vi "HeaderAction.vi"(0 "EG_G5210 en entrée":refnum<class "EGG5210.lvclass"> caption="DNL_LabVIEW Object in", 11 "error in (no error)":errorcluster caption="entrée d'erreur (pas d'erreur)") -> (4 "EG_G5210 en sortie":refnum<class "EGG5210.lvclass"> caption="DNL_LabVIEW Object out", 6 "DataNames":string[](array[string]), 8 "Instr Name":string, 10 "HeaderString":string, 14 "DisplayNames":string[](array[string]), 15 "error out":errorcluster caption="sortie d'erreur")   [LabVIEW 2012, in "EGG5210.lvclass"]
uses:
  EGG5210.lvclass
  EGG5210.lvclass/EGG5210.ctl
  <userlib>/EG_G 5210 LIA/ReadFunctions.ctl
  <userlib>/EG_G 5210 LIA/TrigMode.ctl
  BaseDevice/BaseDevice.lvclass
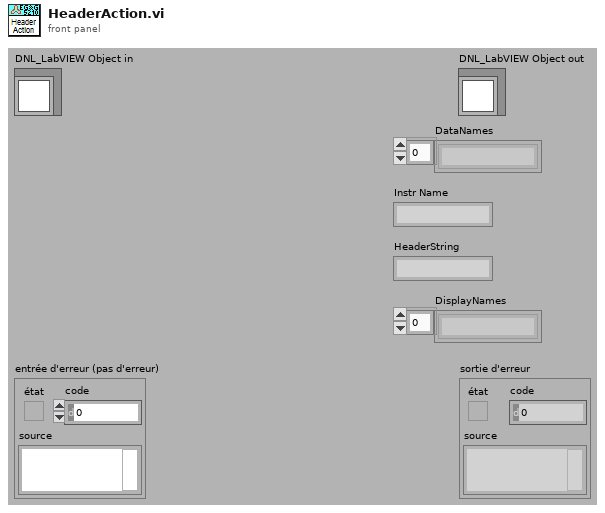
[diagram p1: front panel]
types:
  T1 = typedef "ReadFunctions.ctl" = enum16{"Sensitivity", "Vernier Mode", "Main Filter", "Filter Mode", "Line Filter", "Ref Source", "Ref Mode", "Ref Phase", "Ref Frequency", "Output Filter", "Time Constant", "Dyn Reserve", "X Offset", "Y Offset", "Expand Mode", "Int Oscillator", "Oscillator Freq", "All params", "Overload Byte", "Trigger Mode", "Error"}
  T2 = typedef "EGG5210.lvclass/EGG5210_Func.ctl" = enum16{"Read X & Y (V)", "Read Mag & Phase (V,°)", "Read X, Y, Mag & Phase (V,V,V,°)", "Read ADC Ch1 (V)", "Read ADC Ch2 (V)", "Oscillator Ctrl (Hz, mV rms)", "PL Excimer Settings (Na)"}
  T3 = typedef "TrigMode.ctl" = u16
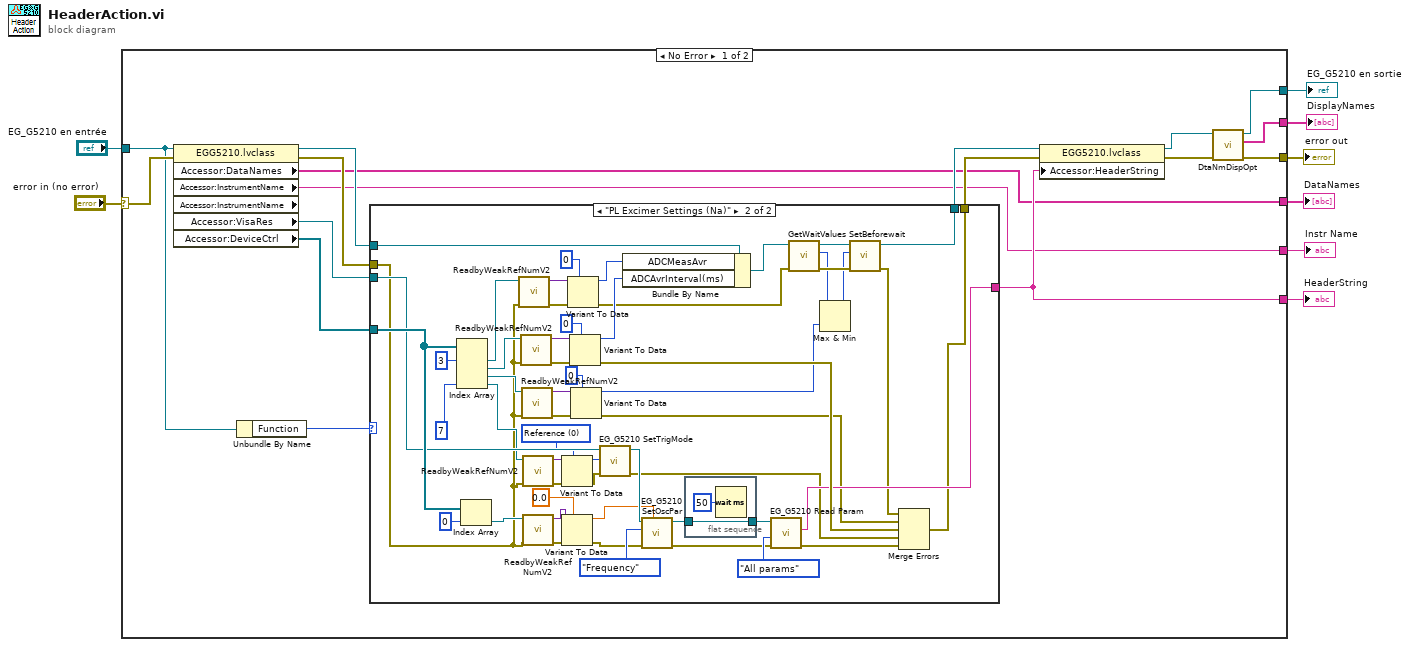
[diagram p0: block diagram]
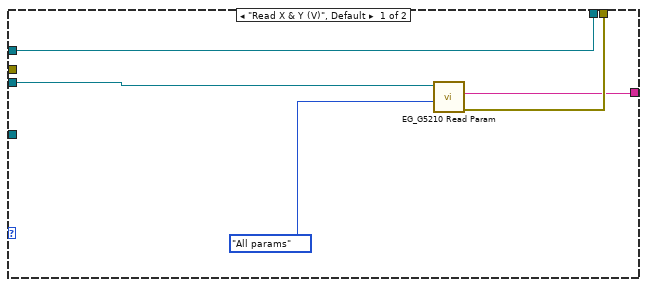
[diagram p2: hidden frame]
diagram:
  n1 = case shown="No Error" "error in (no error)" {
    selector: "error in (no error)" -> [w25 w87]
    tunnel: "EG_G5210 en entrée" -> [w22 w88]
    tunnel: [w10 w88] -> w6
    tunnel: [w15 _] -> w5
    tunnel: [w24 _] -> w4
    tunnel: [w11 w87] -> w3
    tunnel: [w14 _] -> w2
    tunnel: [w9 _] -> w1
    frame No Error {
      n2 = property class="EGG5210.lvclass" props=["Accessor:DataNames", "Accessor:InstrumentName", "Accessor:InstrumentName", "Accessor:VisaRes", "Accessor:DeviceCtrl"](reference=w22, error in=w25) -> (reference out=w16:refnum<class "EGG5210.lvclass">, error out=w17:errorcluster, "Accessor:DataNames"=w15:string[], "Accessor:InstrumentName"=w14:string, "Accessor:VisaRes"=w18:refnum<visa-resource-name>, "Accessor:DeviceCtrl"=w20:refnum<vi>[])  [unwired: 1 out]
      n3 = Unbundle By Name(w22) -> ("Function"=w21:T2)
      n4 = case shown="\"PL Excimer Settings (Na)\"" w21 {
        tunnel: w18 -> [w29 w65]
        tunnel: [w28 w63] -> w24
        tunnel: [w30 w62] -> w23
        tunnel: w20 -> [_ w66]
        tunnel: w16 -> [w26 w64]
        tunnel: [w26 w47] -> w19
        tunnel: w17 -> [_ w35]
        frame "Read X & Y (V)", Default {
          n5 = call <userlib>:"EG_G5210 Read Param.vi"("Énum"=ReadFunctions."All params", "Ressource VISA"=w29) -> ("error out"=w30:errorcluster, "Params"=w28:string)  [unwired: 6 in, 2 out]
        }
        frame "PL Excimer Settings (Na)" {
          w59 = T3 0 items=["Reference", "External", "Asynchronous", "Ratio", "8F"] ("TrigMode")
          n6 = Index Array(array=w66, index #1=3 ("indice"), index #4=7 ("index")) -> (element #1=w80:refnum<vi>, element #2=w84:refnum<vi>, element #3=w36:refnum<vi>, element #4=w40:refnum<vi>)  [unwired: 2 in]
          n7 = Index Array(array=w66, index=0 ("indice")) -> (element=w55:refnum<vi>)
          n8 = call <userlib>:"ReadbyWeakRefNumV2.vi"("error in"=w35, "Control Ref"=w80) -> ("error out"=w74:errorcluster, "Valeur"=w73:variant)  [unwired: 8 in]
          n9 = call <userlib>:"ReadbyWeakRefNumV2.vi"("error in"=w35, "Control Ref"=w84) -> ("error out"=w69:errorcluster, "Valeur"=w70:variant)  [unwired: 8 in]
          n10 = call <userlib>:"ReadbyWeakRefNumV2.vi"("error in"=w35, "Control Ref"=w36) -> ("error out"=w39:errorcluster, "Valeur"=w38:variant)  [unwired: 8 in]
          n11 = call <userlib>:"ReadbyWeakRefNumV2.vi"("error in"=w35, "Control Ref"=w40) -> ("error out"=w60:errorcluster, "Valeur"=w61:variant)  [unwired: 8 in]
          n12 = call <userlib>:"ReadbyWeakRefNumV2.vi"("error in"=w35, "Control Ref"=w55) -> ("error out"=w56:errorcluster, "Valeur"=w54:variant)  [unwired: 8 in]
          n13 = Variant To Data(error in=w60, type=w59, Variant=w61) -> (data=w58:T3, error out=w57:errorcluster)
          n14 = Variant To Data(error in=w56, type=0.0 ("Frequency"), Variant=w54) -> (data=w51:dbl, error out=w53:errorcluster)
          n15 = Variant To Data(error in=w74, type=u32 0 ("indice"), Variant=w73) -> (data=w71:u32, error out=w45:errorcluster)
          n16 = Variant To Data(error in=w69, type=u32 0 ("indice"), Variant=w70) -> (data=w67:u32, error out=w83:errorcluster)
          n17 = Variant To Data(error in=w39, type=u32 0 ("y"), Variant=w38) -> (data=w33:u32, error out=w34:errorcluster)
          n18 = call <userlib>:"EG_G5210 SetTrigMode.vi"("error in (no error)"=w57, "TrigMode"=w58, "Ressource VISA"=w65) -> ("error out"=w50:errorcluster, "Ressource VISA Out"=w76:refnum<visa-resource-name>)  [unwired: 7 in]
          n19 = Bundle By Name(cluster=w64, "ADCMeasAvr"=w71, "ADCAvrInterval(ms)"=w67) -> (w46:refnum<class "EGG5210.lvclass">)
          n20 = call <userlib>:"EG_G5210 SetOscPar.vi"("Frequency"=w51, "error in (no error)"=w53, "Énum"=enum16{"Amplitude", "Frequency"}."Frequency", "Ressource VISA"=w76) -> ("error out"=w78:errorcluster, "Ressource VISA Out"=w48:refnum<visa-resource-name>)  [unwired: 6 in]
          n21 = flat-sequence {
            tunnel: [w86] -> w49
            tunnel: w48 -> [w86]
            frame #0 {
              n22 = Wait (ms)(milliseconds to wait=u32 50) -> ()  [unwired: 1 out]
            }
          }
          n23 = call <userlib>:"EG_G5210 Read Param.vi"("error in (no error)"=w78, "Énum"=ReadFunctions."All params", "Ressource VISA"=w49) -> ("error out"=w82:errorcluster, "Params"=w63:string)  [unwired: 5 in, 2 out]
          n24 = call "GetWaitValues.vi"("error in (no error)"=w45, "BaseDevice en entrée"=w46) -> ("error out"=w44:errorcluster, "Beforewait(ms)"=w42:u32, "BaseDevice en sortie"=w43:refnum<class "EGG5210.lvclass">)  [unwired: 5 in, 2 out]
          n25 = Max & Min(x=w42, y=w33) -> (max(x,y)=w32:u32)  [unwired: 1 out]
          n26 = call "SetBeforewait.vi"("error in (no error)"=w44, "Beforewait(ms)"=w32, "BaseDevice en entrée"=w43) -> ("error out"=w31:errorcluster, "BaseDevice en sortie"=w47:refnum<class "EGG5210.lvclass">)  [unwired: 7 in]
          n27 = Merge Errors(w31, w34, w83, w50, w82) -> (w62:errorcluster)
        }
      }
      n28 = property class="EGG5210.lvclass"(reference=w19, error in=w23, "Accessor:HeaderString"=w24) -> (reference out=w13:refnum<class "EGG5210.lvclass">, error out=w12:errorcluster)
      n29 = call "DtaNmDispOpt.vi"("error in (no error)"=w12, "BaseDevice en entrée"=w13) -> ("error out"=w11:errorcluster, "DisplayNames"=w9:string[], "BaseDevice en sortie"=w10:refnum<class "EGG5210.lvclass">)  [unwired: 7 in]
    }
    frame Error {
    }
  }
  "error out" <- w3
  "EG_G5210 en sortie" <- w6
  "DataNames" <- w5
  "HeaderString" <- w4
  "Instr Name" <- w2
  "DisplayNames" <- w1
